vi "Field Draw Balls.vi"(4 "Draw Targets?":T1, 6 "side":enum16{"Esquerdo", "Direito"}(ring), 8 "Picture In":picture, 9 "Offset":cluster{"Width":dbl, "Height":dbl}, 10 "Scale":dbl, 11 "BallRef":refnum<class "Ball.lvclass">) -> (0 "Picture Out":picture, 1 "Offset Out":cluster{"Width":dbl, "Height":dbl}, 2 "Scale Out":dbl)   [LabVIEW 2018]
uses:
  DrawTargets.ctl
  Ball_class/Ball.lvclass
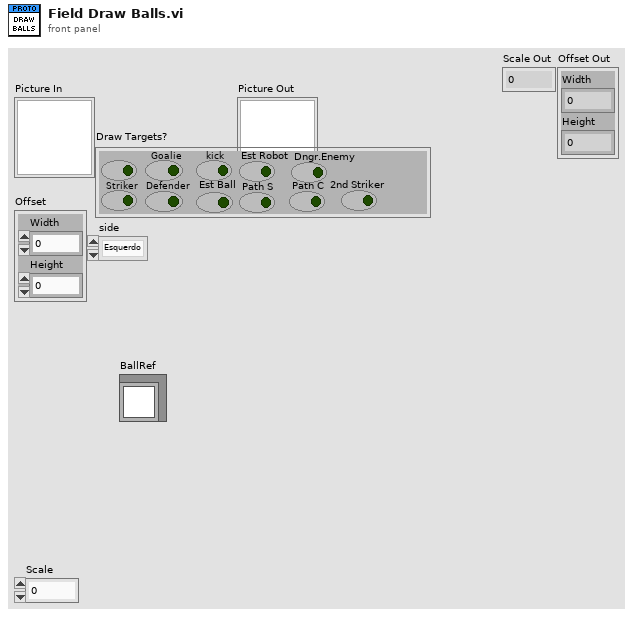
[diagram p1: front panel]
types:
  T1 = typedef "DrawTargets.ctl" = cluster{"Attacker":bool, "Striker":bool, "Goalie":bool, "Defender":bool, "kick":bool, "Est Ball":bool, "Est Robot":bool, "Path S":bool, "Path C":bool, "Dngr.Enemy":bool, "2nd Striker":bool}
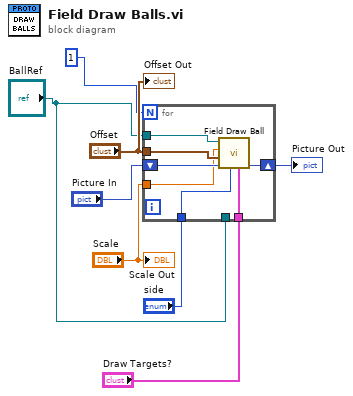
[diagram p0: block diagram]
diagram:
  n1 = for {
    N: 1 -> [_]
    tunnel: "Scale" -> [w11]
    tunnel: "Offset" -> [w12]
    tunnel: "BallRef" -> [w13]
    shift-right: [w15] -> w5
    shift-left: "Picture In" -> [w14]
    tunnel: "BallRef" -> [_]
    tunnel: "Draw Targets?" -> [w10]
    tunnel: "side" -> [w9]
    n2 = call "Field Draw Ball.vi"("Draw Targets?"=w10, "Lado"=w9, "picture in"=w14, "Offset"=w12, "Scale mm/pixel"=w11, "BallRef"=w13) -> ("picture out"=w15:picture)  [unwired: 5 in]
  }
  "Picture Out" <- w5
  "Scale Out" <- "Scale"
  "Offset Out" <- "Offset"
